vi "DefineFileName.vi"(0 "Sample Time":timestamp, 1 "DataFolder":path, 3 "FirstLog?":bool, 5 "error in (no error)":errorcluster) -> (14 "FileName":string, 19 "error out":errorcluster)   [LabVIEW 2014, in "IndoorData.lvclass"]
uses:
  IndoorData.lvclass
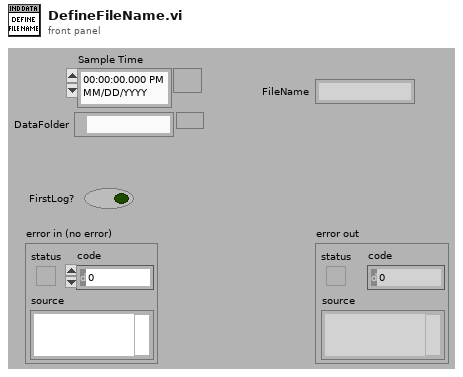
[diagram p1: front panel]
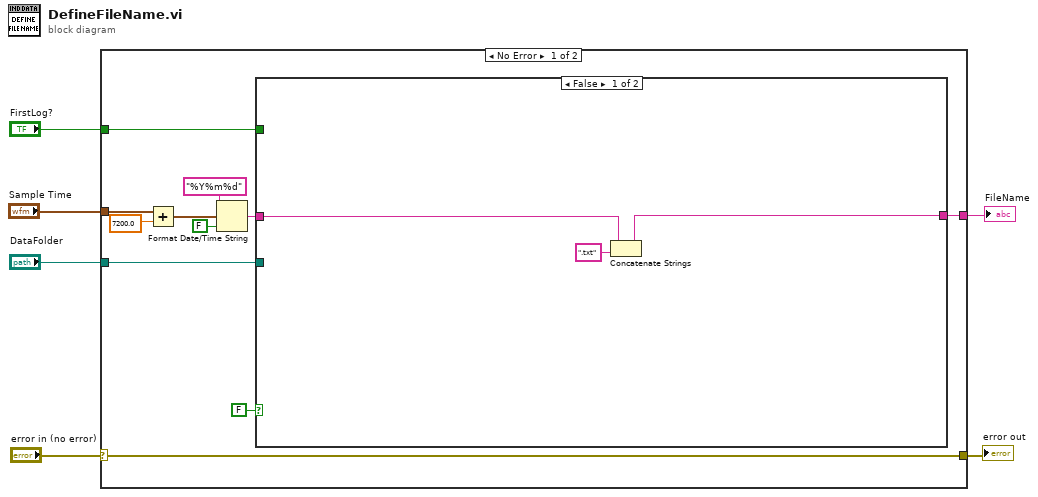
[diagram p0: block diagram]
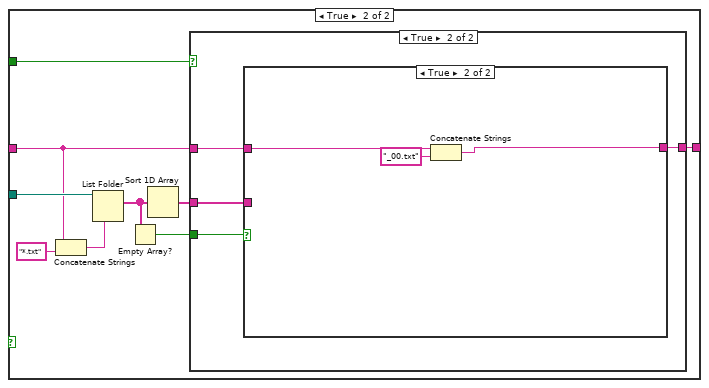
[diagram p2: hidden frame]
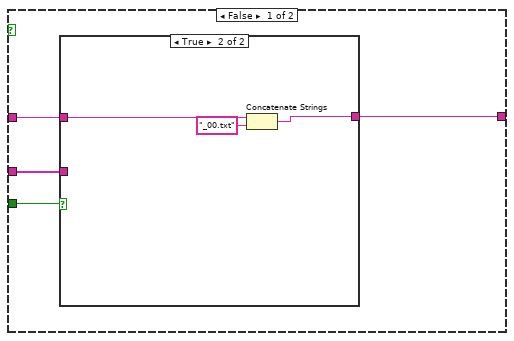
[diagram p3: hidden frame]
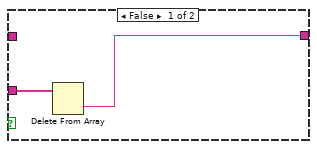
[diagram p4: hidden frame]
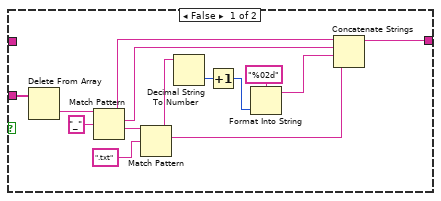
[diagram p5: hidden frame]
diagram:
  n1 = case shown="No Error" "error in (no error)" {
    selector: "error in (no error)" -> [w17 w60]
    tunnel: [w17 w60] -> w5
    tunnel: "DataFolder" -> [w16 _]
    tunnel: "Sample Time" -> [w11 _]
    tunnel: "FirstLog?" -> [w15 _]
    tunnel: [w14 _] -> w1
    frame No Error {
      n2 = Add(x=w11, y=7200.0) -> (x+y=w9:timestamp)
      n3 = Format Date/Time String(time format string (%c)="%Y%m%d", seconds (now)=w9, UTC format=FALSE) -> (date/time string=w8:string)
      n4 = case shown="False" FALSE {
        tunnel: w16 -> [_ w29]
        tunnel: w15 -> [_ w26]
        tunnel: [w18 w23] -> w14
        tunnel: w8 -> [w19 w21]
        frame False {
          n5 = Concatenate Strings(w19, ".txt" ("string")) -> (w18:string)
        }
        frame True {
          n6 = Concatenate Strings(w21, "*.txt" ("string")) -> (w27:string)
          n7 = List Folder(path=w29, pattern=w27) -> (filenames=w24:string[])  [unwired: 2 in, 3 out]
          n8 = Empty Array?(array=w24) -> (empty?=w25:bool)
          n9 = Sort 1D Array(array=w24) -> (sorted array=w22:string[])
          n10 = case shown="True" w26 {
            tunnel: w25 -> [w33 w41]
            tunnel: w21 -> [w32 w40]
            tunnel: w22 -> [w31 w39]
            tunnel: [w30 w42] -> w23
            frame False {
              n11 = case shown="True" w33 {
                tunnel: w32 -> [_ w38]
                tunnel: w31 -> [w35 _]
                tunnel: [w34 w36] -> w30
                frame False {
                  n12 = Delete From Array(array=w35) -> (deleted portion=w34:string)  [unwired: 2 in, 1 out]
                }
                frame True {
                  n13 = Concatenate Strings(w38, "_00.txt" ("string")) -> (w36:string)
                }
              }
            }
            frame True {
              n14 = case shown="True" w41 {
                tunnel: w40 -> [_ w59]
                tunnel: w39 -> [w56 _]
                tunnel: [w48 w57] -> w42
                frame False {
                  n15 = Delete From Array(array=w56) -> (deleted portion=w55:string)  [unwired: 2 in, 1 out]
                  n16 = Match Pattern(string=w55, regular expression="_") -> (before substring=w51:string, match substring=w50:string, after substring=w52:string)  [unwired: 1 in, 1 out]
                  n17 = Match Pattern(string=w52, regular expression=".txt") -> (before substring=w47:string, match substring=w49:string)  [unwired: 1 in, 2 out]
                  n18 = Decimal String To Number(string=w47) -> (number=w46:i32)  [unwired: 2 in, 1 out]
                  n19 = Increment(x=w46) -> (x+1=w45:i32)
                  n20 = Format Into String(format string="%02d", w45) -> (resulting string=w44:string)  [unwired: 2 in, 1 out]
                  n21 = Concatenate Strings(w51, w50, w44, w49) -> (w48:string)
                }
                frame True {
                  n22 = Concatenate Strings(w59, "_00.txt" ("string")) -> (w57:string)
                }
              }
            }
          }
        }
      }
    }
    frame Error {
    }
  }
  "error out" <- w5
  "FileName" <- w1
